vi "Facade 1.vi"(0 "Data In":T5, 2 "Display State In":T3, 3 "Container State":T4) -> (6 "Data Out":T5, 7 "Display State Out":T3, 8 "Action":T2)   [LabVIEW 2016, in "ZebraTable.lvlib" / "XControl 1.xctl"]
uses:
  XControl 1.xctl
  Data 1.ctl
  <vilib>/_xctls/Container State.ctl
  State 1.ctl
  <vilib>/_xctls/Action.ctl
  <vilib>/Utility/miscctls.llb/LVBoundsTypeDef.ctl
  <vilib>/_xctls/XControlSupport.lvlib
panel:
  out "XControl:Container Bounds":T1
  out "ALL vi":string[][](table)
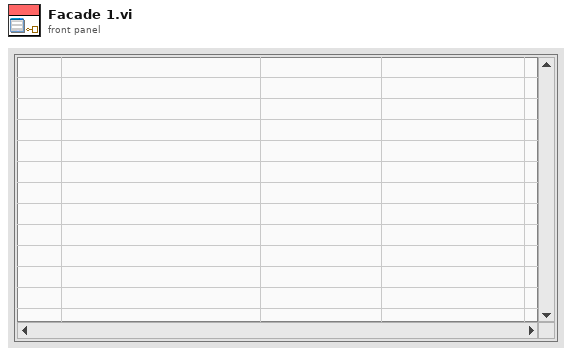
[diagram p1: front panel]
types:
  T1 = typedef "LVBoundsTypeDef.ctl" = cluster{"Width":u32, "Height":u32}
  T2 = typedef "XControlSupport.lvlib/Action.ctl" = cluster{"Data Changed?":bool, "State Changed?":bool, "Action Name":string}
  T3 = typedef "ZebraTable.lvlib/XControl 1.xctl/State 1.ctl" = cluster{"Color Box":u32}
  T4 = typedef "XControlSupport.lvlib/Container State.ctl" = cluster{"Indicator?":bool, "Run Mode?":bool, " Refnum":refnum<vi>}
  T5 = typedef "ZebraTable.lvlib/XControl 1.xctl/Data 1.ctl" = string[][]
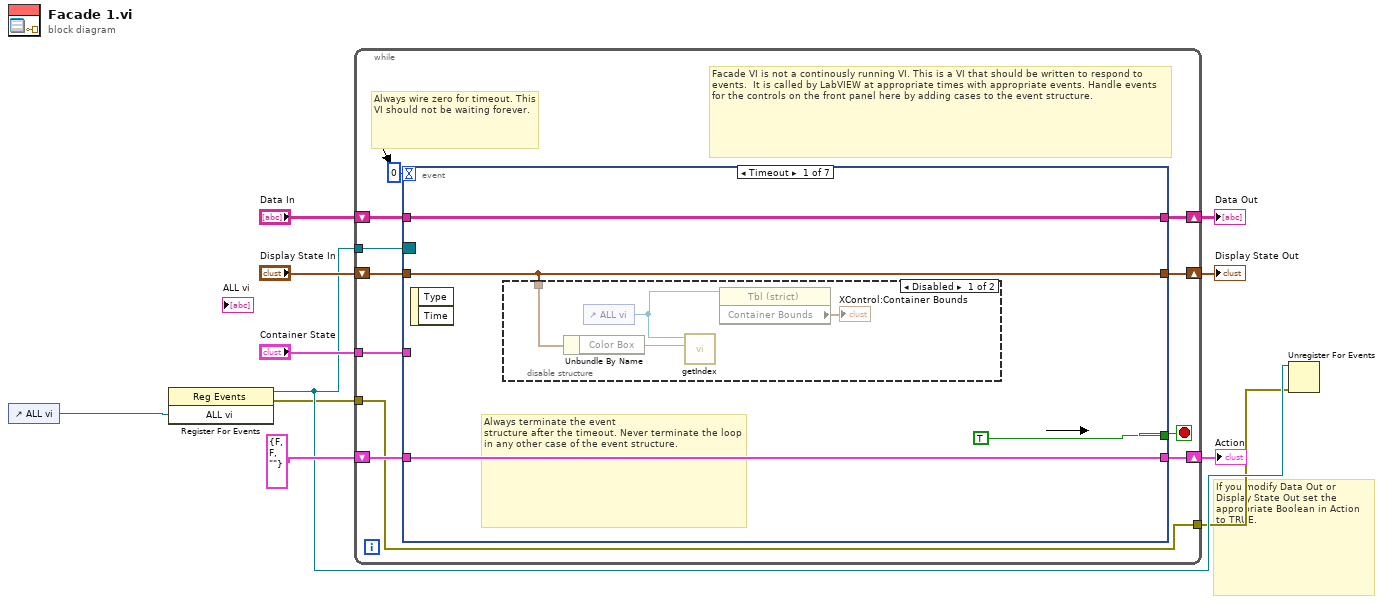
[diagram p0: block diagram]
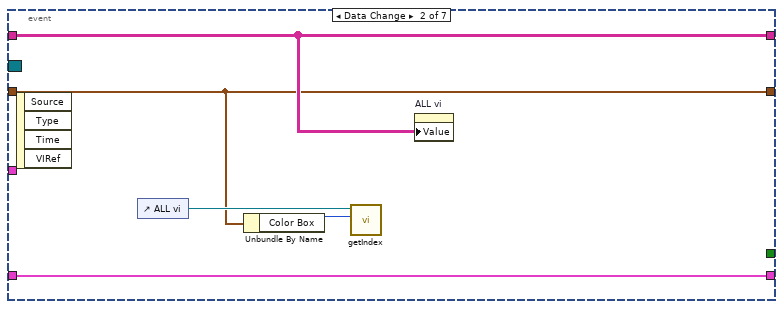
[diagram p3: hidden frame]
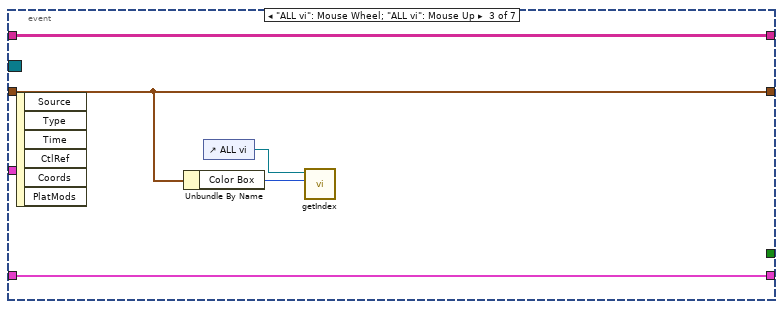
[diagram p4: hidden frame]
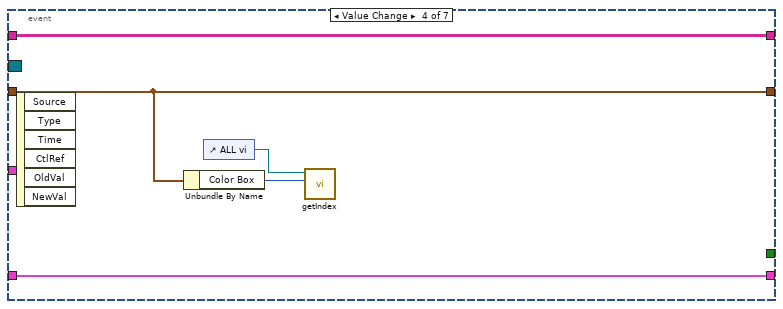
[diagram p5: hidden frame]
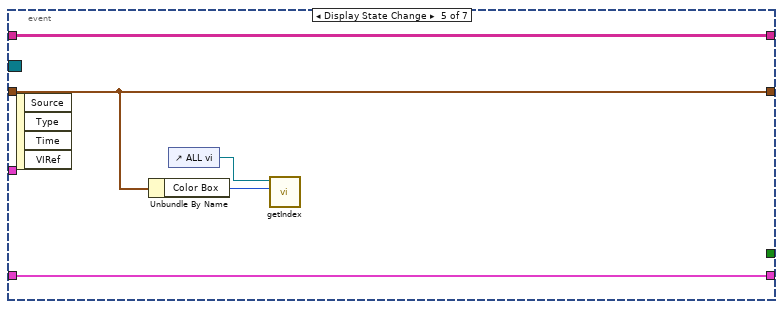
[diagram p6: hidden frame]
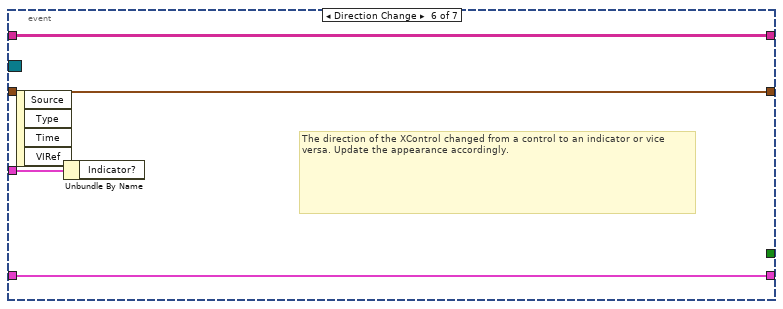
[diagram p7: hidden frame]
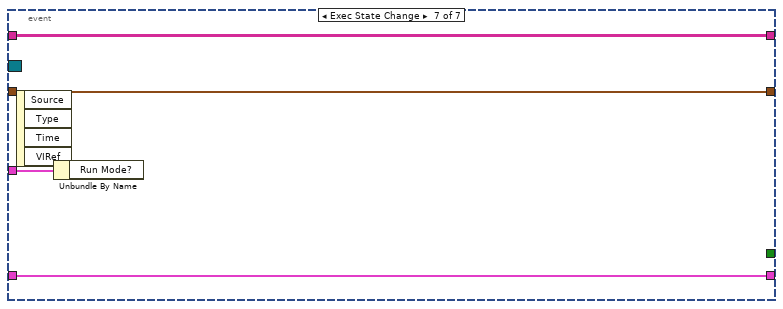
[diagram p8: hidden frame]
diagram:
  # "If you modify Data Out or\nDisplay State Out set the\nappropriate Boolean in Action\nto TRUE."
  n1 = control-ref of="ALL vi"() -> (w2:refnum<vi>)
  n2 = register-events(w2) -> (reference out=w5:refnum<event-registration>, error out=w4:errorcluster)  [unwired: 2 in]
  n3 = while {
    shift-right: [w21] -> w9
    shift-left: "Display State In" -> [w22]
    tunnel: "Container State" -> [w18]
    shift-right: [w16] -> w11
    shift-left: "Data In" -> [w17]
    shift-right: [w14] -> w7
    shift-left: T2 {"Data Changed?"=FALSE, "State Changed?"=FALSE, "Action Name"=""} ("Action") -> [w15]
    tunnel: w5 -> [w13]
    tunnel: [w12] -> w3
    tunnel: w4 -> [w12]
    stop <- w20 stop-if-true
    # "Facade VI is not a continously running VI. This is a VI that should be written to respond to events.  It is called by LabVIEW at appropriate times with appropriate events. Handle events for the controls on the front panel here by adding cases to the event structure."
    # "Always wire zero for timeout. This\nVI should not be waiting forever."
    n4 = event shown="[0] Timeout" {
      selector: w13 -> [_ _ _ _ _ _ _]
      dyn-events: _ -> [_ _ _ _ _ _ _]
      timeout: 0 -> [_ _ _ _ _ _ _]
      tunnel: w22 -> [w24 w32 w38 w43 w48 w53 w55]
      tunnel: [w24 w32 w38 w43 w48 w53 w55] -> w21
      tunnel: [TRUE _ _ _ _ _ _] -> w20
      tunnel: w18 -> [_ _ _ _ _ w54 w58]
      tunnel: w17 -> [w23 w33 w39 w44 w50 w52 w57]
      tunnel: [w23 w33 w39 w44 w50 w52 w57] -> w16
      tunnel: [w25 w35 w40 w45 w49 w51 w56] -> w14
      tunnel: w15 -> [w25 w35 w40 w45 w49 w51 w56]
      event Timeout {
        # "Always terminate the event\nstructure after the timeout. Never terminate the loop in any other case of the event structure."
        n5 = event-data() -> ()  [unwired: 1 in, 2 out]
        n6 = disable-structure shown="Disabled" {
          disable-tunnel: w24 -> [w29 _]
          frame Disabled {
            n7 = Unbundle By Name(w29) -> ("Color Box"=w30:u32)
            n8 = control-ref of="ALL vi"() -> (w28:refnum<vi>)
            n9 = call "getIndex.vi"("Active Cell:Cell Background Color"=w30, "TableRef"=w28) -> ()  [unwired: 9 in, 1 out]
            n10 = property class="Tbl (strict)"(reference=w28) -> ("Container Bounds"=→"XControl:Container Bounds":T1)  [unwired: 1 in, 2 out]
          }
          frame Enabled {
          }
        }
      }
      event Data Change {
        n11 = event-data() -> ()  [unwired: 1 in, 4 out]
        n12 = control-ref of="ALL vi"() -> (w34:refnum<vi>)
        n13 = Unbundle By Name(w32) -> ("Color Box"=w31:u32)
        n14 = call "getIndex.vi"("Active Cell:Cell Background Color"=w31, "TableRef"=w34) -> ()  [unwired: 9 in, 1 out]
        n15 = property on="ALL vi" class="Tbl (strict)"("Value"=w33) -> ()  [unwired: 2 in, 2 out]
      }
      event "ALL vi": Mouse Wheel; "ALL vi": Mouse Up {
        n16 = event-data() -> ()  [unwired: 1 in, 6 out]
        n17 = Unbundle By Name(w38) -> ("Color Box"=w36:u32)
        n18 = control-ref of="ALL vi"() -> (w37:refnum<vi>)
        n19 = call "getIndex.vi"("Active Cell:Cell Background Color"=w36, "TableRef"=w37) -> ()  [unwired: 9 in, 1 out]
      }
      event Value Change {
        n20 = event-data() -> ()  [unwired: 1 in, 6 out]
        n21 = Unbundle By Name(w43) -> ("Color Box"=w41:u32)
        n22 = control-ref of="ALL vi"() -> (w42:refnum<vi>)
        n23 = call "getIndex.vi"("Active Cell:Cell Background Color"=w41, "TableRef"=w42) -> ()  [unwired: 9 in, 1 out]
      }
      event Display State Change {
        n24 = event-data() -> ()  [unwired: 1 in, 4 out]
        n25 = Unbundle By Name(w48) -> ("Color Box"=w46:u32)
        n26 = control-ref of="ALL vi"() -> (w47:refnum<vi>)
        n27 = call "getIndex.vi"("Active Cell:Cell Background Color"=w46, "TableRef"=w47) -> ()  [unwired: 9 in, 1 out]
      }
      event Direction Change {
        # "The direction of the XControl changed from a control to an indicator or vice versa. Update the appearance accordingly."
        n28 = event-data() -> ()  [unwired: 1 in, 4 out]
        n29 = Unbundle By Name(w54) -> ()  [unwired: 1 out]
      }
      event Exec State Change {
        n30 = event-data() -> ()  [unwired: 1 in, 4 out]
        n31 = Unbundle By Name(w58) -> ()  [unwired: 1 out]
      }
    }
  }
  "Display State Out" <- w9
  "Data Out" <- w11
  "Action" <- w7
  n32 = Unregister For Events(event registration refnum=w5, error in=w3) -> ()  [unwired: 1 out]
